vi "Get Application Path.vi"() -> (0 "application path":path)   [LabVIEW 2013]
doc: "When this VI executes, it always returns the name of the main folder, whether it was called from the built executable or from one of the source VIs.\n\nThis VI returns the folder containing the calling VI or .EXE file, UNLESS one of the folder names in the path is \"source\". In that case, it uses the folder one above the source folder. \n\nExplanation: This VI is meant for the standard SFIS folder naming convention. The main folder is often named for the customer or the project. Inside this folder is the EXE file for the build labview application. This main folder can also contain a folder called \"source\" at the next level down. The source folder can contain many subfolders at mutiple levels."
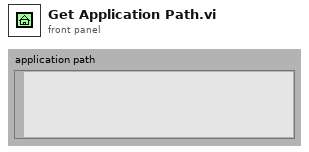
[diagram p1: front panel]
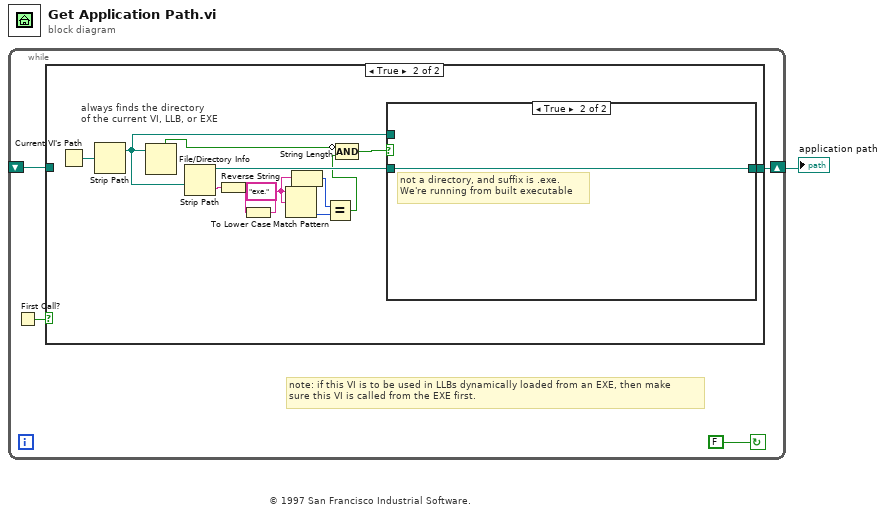
[diagram p0: block diagram]
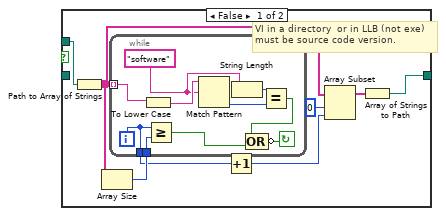
[diagram p3: hidden frame]
diagram:
  # "© 1997 San Francisco Industrial Software."
  n1 = while {
    shift-left: _ -> [w4]
    shift-right: [w5] -> w1
    stop <- FALSE continue-if-true
    # "note: if this VI is to be used in LLBs dynamically loaded from an EXE, then make\nsure this VI is called from the EXE first."
    n2 = First Call?() -> (First Call?: T/F=w2:bool)
    n3 = case shown="True" w2 {
      tunnel: [w6 w19] -> w5
      tunnel: w4 -> [w6 _]
      frame False {
      }
      frame True {
        w11 = "exe." ("regular expression")
        # "always finds the directory\nof the current VI, LLB, or EXE"
        n4 = Current VI's Path() -> (path=w7:path)
        n5 = Strip Path(path=w7) -> (stripped path=w8:path)  [unwired: 1 out]
        n6 = File/Directory Info(path=w8) -> (directory=w18:bool)  [unwired: 1 in, 6 out]
        n7 = Strip Path(path=w8) -> (stripped path=w17:path, name=w13:string)
        n8 = Reverse String(1:w13) -> (0:w12:string)
        n9 = To Lower Case(string=w12) -> (all lower case string=w14:string)
        n10 = Match Pattern(string=w14, regular expression=w11) -> (offset past match=w15:i32)  [unwired: 1 in, 3 out]
        n11 = String Length(string=w11) -> (length=w10:i32)
        n12 = Equal?(x=w10, y=w15) -> (x = y?=w9:bool)
        n13 = Compound Arithmetic op=AND(invert w18, w9) -> (w16:bool)
        n14 = case shown="True" w16 {
          tunnel: w8 -> [w27 _]
          tunnel: w17 -> [_ w38]
          tunnel: [w22 w38] -> w19
          frame False {
            # "VI in a directory  or in LLB (not exe)\nmust be source code version."
            n15 = Path to Array of Strings(0:w27) -> (2:w26:string[])  [unwired: 1 out]
            n16 = Array Size(array=w26) -> (size(s)=w25:i32)
            n17 = while {
              tunnel: [w30] -> w24
              tunnel: w25 -> [w32]
              tunnel: w26 -> [w36] mode=indexing
              i -> [w30]
              stop <- w35 continue-if-true
              w29 = "software"
              n18 = To Lower Case(string=w36) -> (all lower case string=w37:string)
              n19 = Greater Or Equal?(x=w30, y=w32) -> (x >= y?=w31:bool)
              n20 = Match Pattern(string=w37, regular expression=w29) -> (offset past match=w34:i32)  [unwired: 1 in, 3 out]
              n21 = String Length(string=w29) -> (length=w28:i32)
              n22 = Equal?(x=w28, y=w34) -> (x = y?=w33:bool)
              n23 = Compound Arithmetic op=OR(w33, w31) -> (invert w35:bool)
            }
            n24 = Increment(x=w24) -> (x+1=w20:i32)
            n25 = Array Subset(array=w26, index=0, length=w20) -> (w21:string[])
            n26 = Array of Strings to Path(0:w21) -> (2:w22:path)  [unwired: 1 in]
          }
          frame True {
            # "not a directory, and suffix is .exe.\nWe're running from built executable"
          }
        }
      }
    }
  }
  "application path" <- w1
